vi "Panel Actor Event Loop.vi"   [LabVIEW 2023]
doc: "Drops a basic template Event Handler Loop that is useful for Panel Actors.\n\n----\nPlease see the following web address for additional documentation and tutorial information:\nhttp://www.mooregoodideas.com/mgi-panel-manager/\n\nAuthor: Derek Trepanier\n\nCopyright (c) 2018, Moore Good Ideas, Inc.\n\nAll rights reserved.\n\nRedistribution and use in source and binary forms, with or without modification, are permitted provided that the following conditions are met:\n\n * Redistributions of source code must retain the above copyright notice, this list of conditions and the following disclaimer.\n * Redistributions in binary form must reproduce the above copyright notice, this list of conditions and the following disclaimer in the documentation and/or other materials provided with the distribution.\n * Neither the name of Moore Good Ideas, Inc. nor the names of its contributors may be used to endorse or promote products derived from this software without specific prior written permission.\n\nTHIS SOFTWARE IS PROVIDED BY THE COPYRIGHT HOLDERS AND CONTRIBUTORS \"AS IS\" AND ANY EXPRESS OR IMPLIED WARRANTIES, INCLUDING, BUT NOT LIMITED TO, THE IMPLIED WARRANTIES OF MERCHANTABILITY AND FITNESS FOR A PARTICULAR PURPOSE ARE DISCLAIMED. IN NO EVENT SHALL THE COPYRIGHT OWNER OR CONTRIBUTORS BE LIABLE FOR ANY DIRECT, INDIRECT, INCIDENTAL, SPECIAL, EXEMPLARY, OR CONSEQUENTIAL DAMAGES (INCLUDING, BUT NOT LIMITED TO, PROCUREMENT OF SUBSTITUTE GOODS OR SERVICES; LOSS OF USE, DATA, OR PROFITS; OR BUSINESS INTERRUPTION) HOWEVER CAUSED AND ON ANY THEORY OF LIABILITY, WHETHER IN CONTRACT, STRICT LIABILITY, OR TORT (INCLUDING NEGLIGENCE OR OTHERWISE) ARISING IN ANY WAY OUT OF THE USE OF THIS SOFTWARE, EVEN IF ADVISED OF THE POSSIBILITY OF SUCH DAMAGE."
uses:
  <vilib>/ActorFramework/Stop Msg/Stop Msg.lvclass
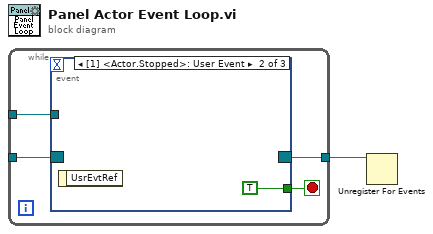
[diagram p0: block diagram]
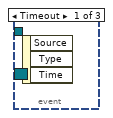
[diagram p2: hidden frame]
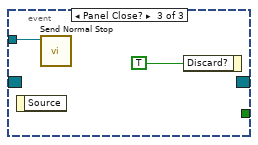
[diagram p3: hidden frame]
diagram:
  n1 = while {
    tunnel: _ -> [w5]
    tunnel: _ -> [w4]
    tunnel: [w2] -> w1
    stop <- w3 stop-if-true
    n2 = event shown="[1] <Actor.Stopped>: User Event" {
      selector: w5 -> [_ _ _]
      dyn-events: [_ _ _] -> w2
      timeout: _ -> [_ _ _]
      tunnel: w4 -> [_ _ w8]
      tunnel: [_ TRUE _] -> w3
      event Timeout {
        n3 = event-data() -> ()  [unwired: 1 in, 3 out]
      }
      event User Event {
        n4 = event-data() -> ()  [unwired: 1 in, 1 out]
      }
      event Panel Close? {
        n5 = event-data() -> ()  [unwired: 1 in, 1 out]
        n6 = call <vilib>:"Send Normal Stop.vi"("Message Enqueuer"=w8) -> ()  [unwired: 10 in, 1 out]
        n7 = event-data("Discard?"=TRUE) -> ()  [unwired: 1 in, 1 out]
      }
    }
  }
  n8 = Unregister For Events(event registration refnum=w1) -> ()  [unwired: 1 in, 1 out]
